vi "Break down Sensor String.vi"(8 "Error in":errorcluster, 11 "Input String":string) -> (0 "Error Out":errorcluster, 3 "Output":string[](array[string]))   [LabVIEW 2016, in "Vires VTD System Explorer.lvlib"]
uses:
  <vilib>/regexp/Match Regular Expression.xnode
  Vires VTD System Explorer.lvlib
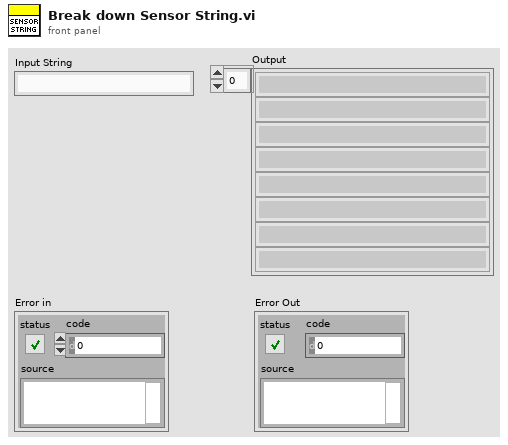
[diagram p1: front panel]
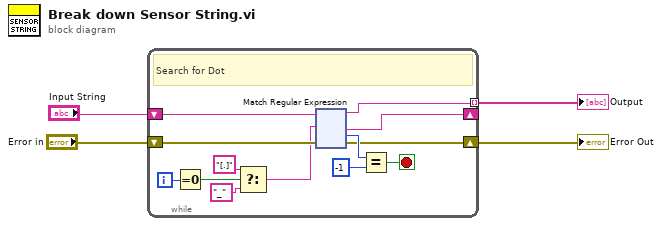
[diagram p0: block diagram]
diagram:
  n1 = while {
    shift-right: [w16] -> _
    shift-left: "Input String" -> [w17]
    tunnel: [w15] -> w1 mode=indexing
    shift-right: [w10] -> w2
    shift-left: "Error in" -> [w11]
    i -> [w9]
    stop <- w12 stop-if-true
    # "Search for Dot"
    n2 = Equal To 0?(x=w9) -> (x = 0?=w8:bool)
    n3 = Select(t="[.]" ("regular expression"), s=w8, f="_" ("regular expression")) -> (s? t:f=w5:string)
    n4 = xnode "Match Regular Expression"("input string"=w17, "regular expression"=w5, "error in"=w11) -> ("before match"=w15:string, "after match"=w16:string, "offset past match"=w14:i32, "error out"=w10:errorcluster)  [unwired: 3 in, 1 out]
    n5 = Equal?(x=w14, y=-1) -> (x = y?=w12:bool)
  }
  "Output" <- w1
  "Error Out" <- w2
